vi "scientific calculator.vi"() -> ()   [LabVIEW 2016]
panel:
  in  "CLR":bool
  out "CALCULATOR":string
  in  "?":T1
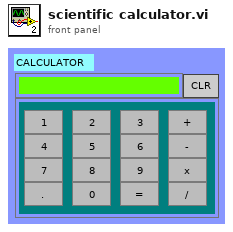
[diagram p1: front panel]
types:
  T1 = cluster{"1":bool, "4":bool, " 2":bool, "3":bool, "5":bool, "6":bool, "7":bool, "8":bool, "=":bool, "0":bool, "+":bool, "-":bool, "x":bool, "/":bool, "9":bool, ".":bool}
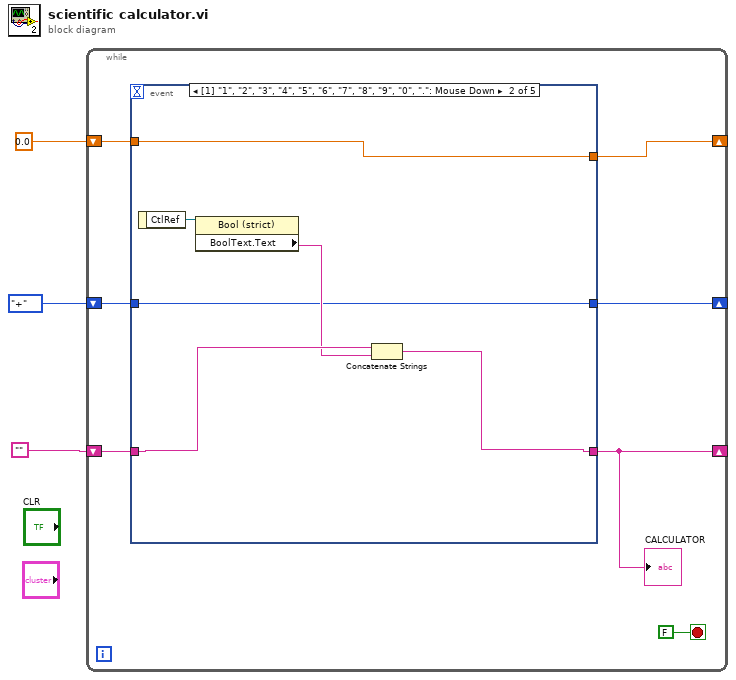
[diagram p0: block diagram]
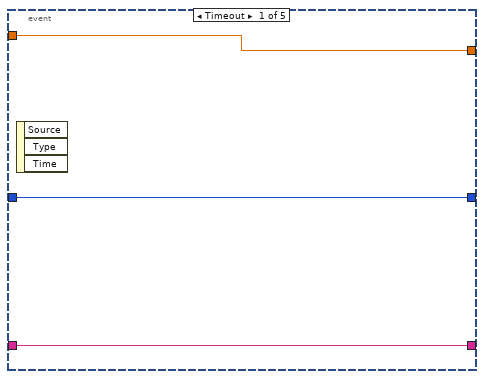
[diagram p2: hidden frame]
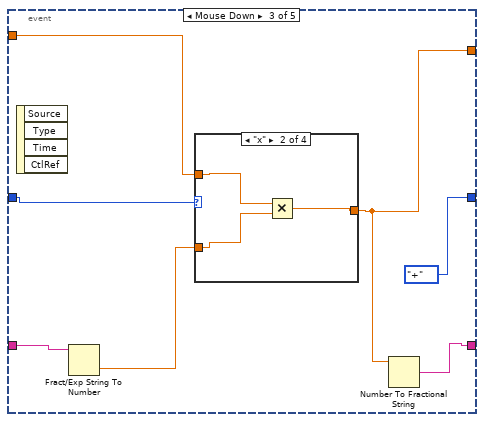
[diagram p3: hidden frame]
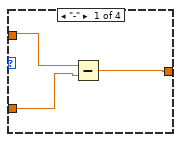
[diagram p4: hidden frame]
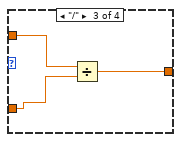
[diagram p5: hidden frame]
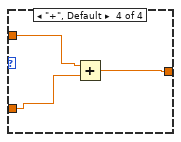
[diagram p6: hidden frame]
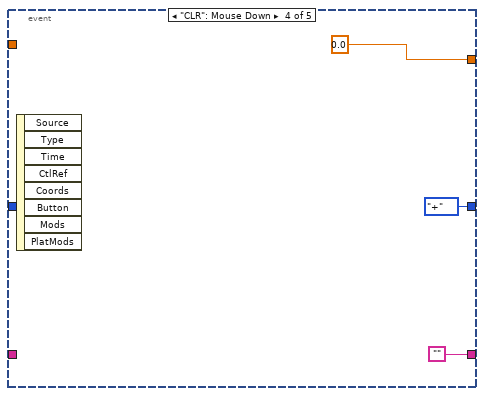
[diagram p7: hidden frame]
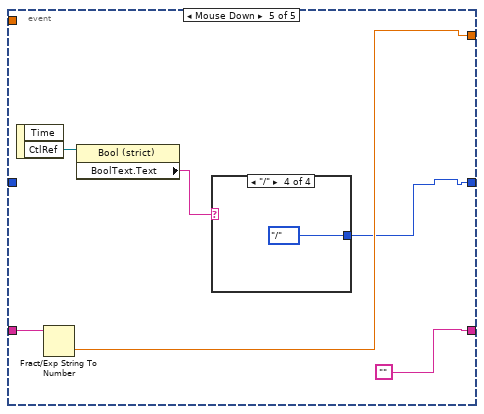
[diagram p8: hidden frame]
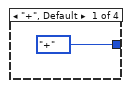
[diagram p9: hidden frame]
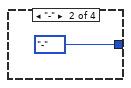
[diagram p10: hidden frame]
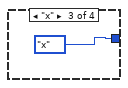
[diagram p11: hidden frame]
diagram:
  n1 = while {
    shift-right: [w6] -> _
    shift-left: 0.0 -> [w7]
    shift-right: [w8] -> _
    shift-left: enum16{"-", "+", "x", "/"}."+" -> [w9]
    shift-right: [w4] -> _
    shift-left: "" -> [w5]
    stop <- FALSE stop-if-true
    n2 = event shown="[1] \"1\", \"2\", \"3\", \"4\", \"5\", \"6\", \"7\", \"8\", \"9\", \"0\", \".\": Mouse Down" {
      selector: _ -> [_ _ _ _ _]
      dyn-events: _ -> [_ _ _ _ _]
      timeout: _ -> [_ _ _ _ _]
      tunnel: [w13 w15 enum16{"-", "+", "x", "/"}."+" enum16{"-", "+", "x", "/"}."+" w43] -> w8
      tunnel: w9 -> [w13 w15 w25 _ _]
      tunnel: w7 -> [w12 w14 w24 _ _]
      tunnel: [w12 w14 w22 0.0 w46] -> w6
      tunnel: w5 -> [w11 w18 w26 _ w47]
      tunnel: [w11 w16 w21 "" ""] -> w4
      event Timeout {
        n3 = event-data() -> ()  [unwired: 1 in, 3 out]
      }
      event Mouse Down {
        n4 = event-data() -> ("CtlRef"=w19:refnum<vi>)  [unwired: 1 in]
        n5 = property class="Bool (strict)"(reference=w19) -> ("BoolText.Text"=w17:string)  [unwired: 1 in, 2 out]
        n6 = Concatenate Strings(w18, w17) -> (w16:string)
      }
      event Mouse Down {
        n7 = event-data() -> ()  [unwired: 1 in, 4 out]
        n8 = Fract/Exp String To Number(string=w26) -> (number=w23:dbl)  [unwired: 3 in, 1 out]
        n9 = case shown="\"x\"" w25 {
          tunnel: w24 -> [w29 w32 w35 w38]
          tunnel: w23 -> [w28 w31 w34 w37]
          tunnel: [w27 w30 w33 w36] -> w22
          frame "-" {
            n10 = Subtract(x=w29, y=w28) -> (x-y=w27:dbl)
          }
          frame "x" {
            n11 = Multiply(x=w32, y=w31) -> (x*y=w30:dbl)
          }
          frame "/" {
            n12 = Divide(x=w35, y=w34) -> (x/y=w33:dbl)
          }
          frame "+", Default {
            n13 = Add(x=w38, y=w37) -> (x+y=w36:dbl)
          }
        }
        n14 = Number To Fractional String(number=w22) -> (F-format string=w21:string)  [unwired: 3 in]
      }
      event "CLR": Mouse Down {
        n15 = event-data() -> ()  [unwired: 1 in, 8 out]
      }
      event Mouse Down {
        n16 = event-data() -> ("CtlRef"=w45:refnum<vi>)  [unwired: 1 in, 1 out]
        n17 = Fract/Exp String To Number(string=w47) -> (number=w46:dbl)  [unwired: 3 in, 1 out]
        n18 = property class="Bool (strict)"(reference=w45) -> ("BoolText.Text"=w44:string)  [unwired: 1 in, 2 out]
        n19 = case shown="\"/\"" w44 {
          tunnel: [enum16{"-", "+", "x", "/"}."+" enum16{"-", "+", "x", "/"}."-" enum16{"-", "+", "x", "/"}."x" enum16{"-", "+", "x", "/"}."/"] -> w43
          frame "+", Default {
          }
          frame "-" {
          }
          frame "x" {
          }
          frame "/" {
          }
        }
      }
    }
    "CALCULATOR" <- w4
  }
